vi "Apply Control Changes.vi"(7 "Type":enum16{"Control", "Indicator"}(ring), 9 "new":string[][](array[string]), 10 "old":string[][](array[string]), 11 "Data In":T1[](array[typedef])) -> (1 "Changed indices":i32[](array[numeric]), 3 "Data Out":T1[](array[typedef]))   [LabVIEW 2023, in "VI Properties Editor.lvlib"]
uses:
  VI Properties Editor.lvlib
  Cluster Data.ctl
  <vilib>/picture/picture.llb/imagedata.ctl
panel:
  # "Connector Pane"
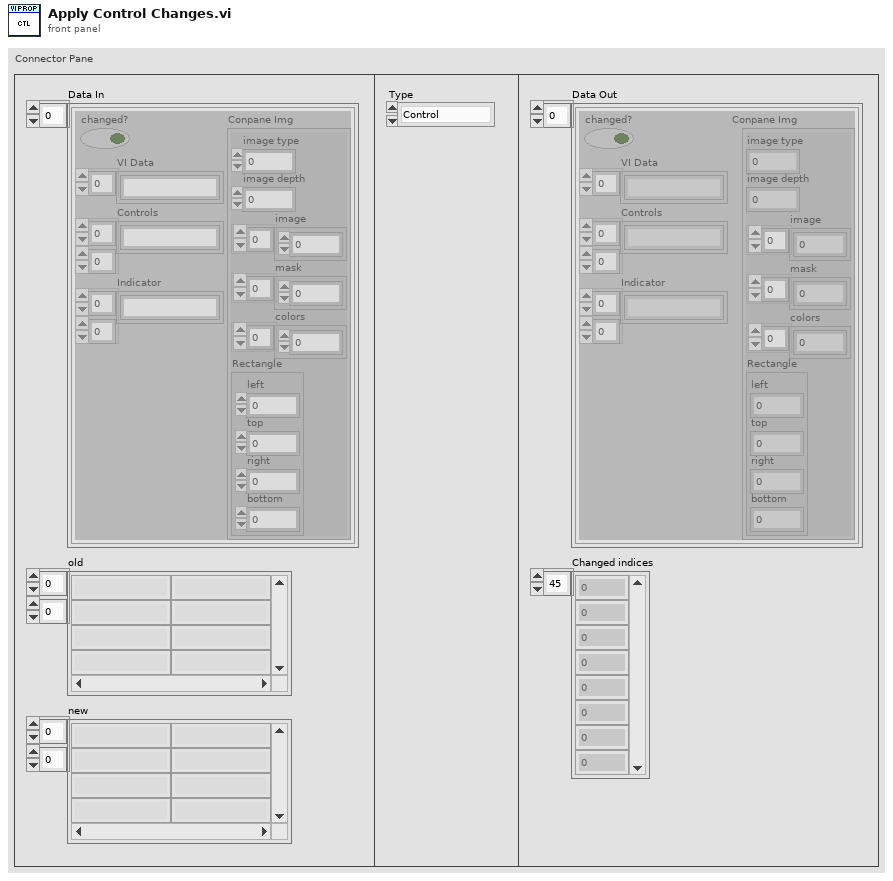
[diagram p1: front panel]
types:
  T1 = typedef "VI Properties Editor.lvlib/Cluster Data.ctl" = cluster{"changed?":bool, "VI Data":string[], "Controls":string[][], "Indicator":string[][], "Conpane Img":T2}
  T2 = typedef "imagedata.ctl" = cluster{"image type":i32, "image depth":i32, "image":u8[], "mask":u8[], "colors":u32[], "Rectangle":cluster{"left":i16, "top":i16, "right":i16, "bottom":i16}}
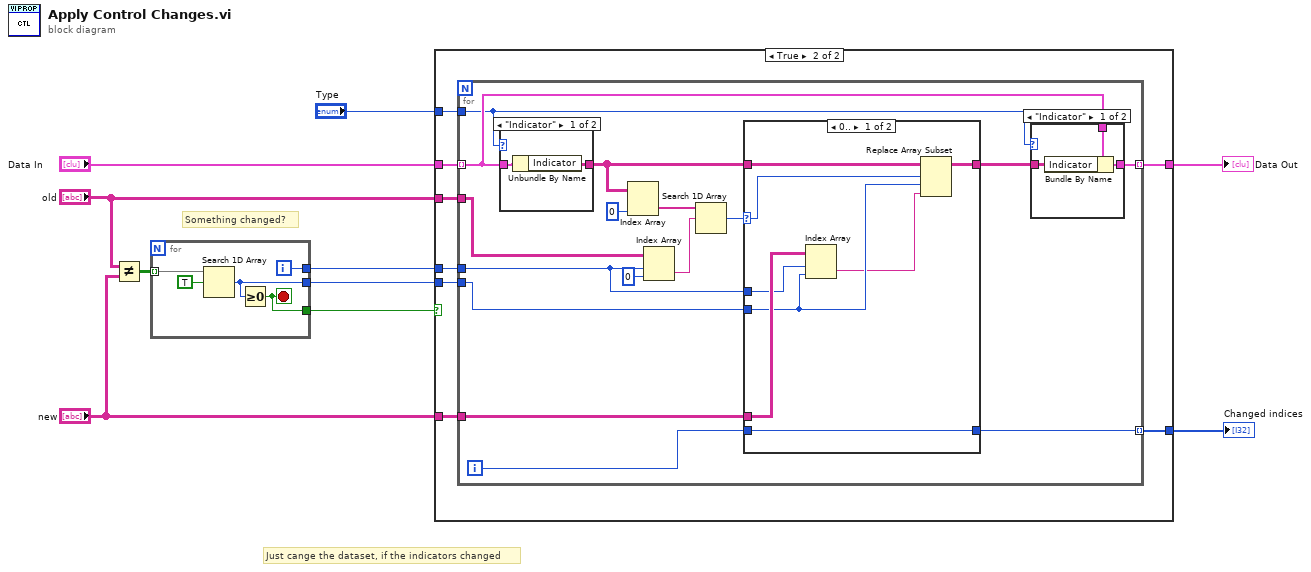
[diagram p0: block diagram]
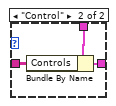
[diagram p3: hidden frame]
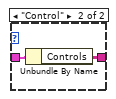
[diagram p4: hidden frame]
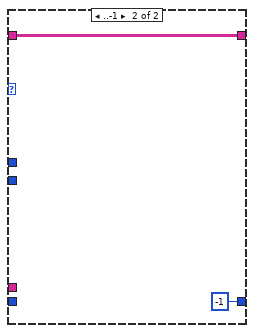
[diagram p5: hidden frame]
diagram:
  # "Just cange the dataset, if the indicators changed"
  # "Something changed?"
  n1 = Not Equal?(x="old", y="new") -> (x != y?=w10:bool[][])
  n2 = for {
    tunnel: w10 -> [w15] mode=indexing
    tunnel: [w13] -> w5
    tunnel: [w12] -> w6
    tunnel: [w11] -> w2
    i -> [w12]
    stop <- w11 stop-if-true
    n3 = Search 1D Array(1D array=w15, element=TRUE) -> (index of element=w13:i32)  [unwired: 1 in]
    n4 = Greater Or Equal To 0?(x=w13) -> (x >= 0?=w11:bool)
  }
  n5 = case shown="True" w2 {
    tunnel: "Data In" -> [w16 w24]
    tunnel: [w16 w20] -> w8
    tunnel: "old" -> [_ w23]
    tunnel: w6 -> [_ w22]
    tunnel: w5 -> [_ w21]
    tunnel: "new" -> [_ w19]
    tunnel: [_ w18] -> w3
    tunnel: "Type" -> [_ w17]
    frame False {
    }
    frame True {
      n6 = for {
        tunnel: w24 -> [w28] mode=indexing
        tunnel: w23 -> [w38]
        tunnel: w22 -> [w32]
        tunnel: w21 -> [w34]
        tunnel: [w26] -> w20 mode=indexing
        tunnel: w19 -> [w33]
        tunnel: [w31] -> w18 mode=indexing
        tunnel: w17 -> [w25]
        i -> [w30]
        n7 = case shown="\"Indicator\"" w25 {
          tunnel: [w48 w50] -> w29
          tunnel: w28 -> [w47 w49]
          frame "Indicator" {
            n8 = Unbundle By Name(w47) -> ("Indicator"=w48:string[][])
          }
          frame "Control" {
            n9 = Unbundle By Name(w49) -> ("Controls"=w50:string[][])
          }
        }
        n10 = Index Array(array=w29, index (col)=0 ("disabled index (col)")) -> (element=w37:string[])  [unwired: 1 in]
        n11 = Index Array(array=w38, index (row)=w32, index (col)=0 ("disabled index (col)")) -> (element=w36:string)
        n12 = Search 1D Array(1D array=w37, element=w36) -> (index of element=w35:i32)  [unwired: 1 in]
        n13 = case shown="0.." w35 {
          selector: w35 -> [w52 _]
          tunnel: w29 -> [w58 w60]
          tunnel: [w57 w60] -> w27
          tunnel: w34 -> [w54 _]
          tunnel: w33 -> [w56 _]
          tunnel: w32 -> [w55 _]
          tunnel: [w51 -1 ("index of element")] -> w31
          tunnel: w30 -> [w51 _]
          frame 0.. {
            n14 = Index Array(array=w56, index (row)=w55, index (col)=w54) -> (element=w53:string)
            n15 = Replace Array Subset(array=w58, new element=w53, index (row)=w52, index (col)=w54) -> (w57:string[][])
          }
          frame ..-1 {
          }
        }
        n16 = case shown="\"Indicator\"" w25 {
          tunnel: w28 -> [w43 w46]
          tunnel: w27 -> [w42 w45]
          tunnel: [w41 w44] -> w26
          frame "Indicator" {
            n17 = Bundle By Name(cluster=w43, "Indicator"=w42) -> (w41:T1)
          }
          frame "Control" {
            n18 = Bundle By Name(cluster=w46, "Controls"=w45) -> (w44:T1)
          }
        }
      }
    }
  }
  "Data Out" <- w8
  "Changed indices" <- w3
